vi "lockin ID.vi"(5 "Addresses IN":refnum<visa-resource-name>[](array[refnum]), 7 "names in":string[](array[string]), 8 "error in (no error)":errorcluster, 9 "Lockin address":string, 10 "Lockin on":bool, 11 "Lockin Chan name":string) -> (0 "error out":errorcluster, 2 "Addresses out":refnum<visa-resource-name>[](array[refnum]), 3 "names out":string[](array[string]))   [LabVIEW 2024]
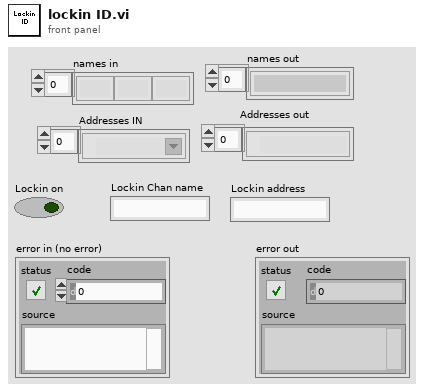
[diagram p1: front panel]
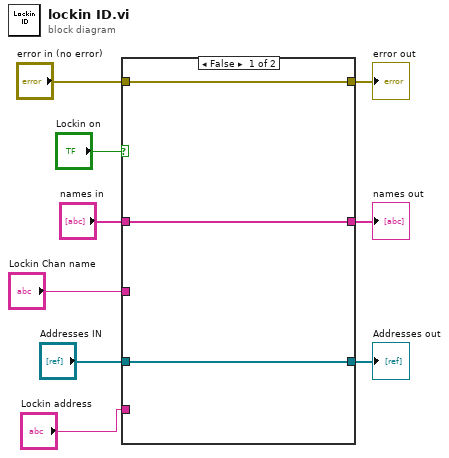
[diagram p0: block diagram]
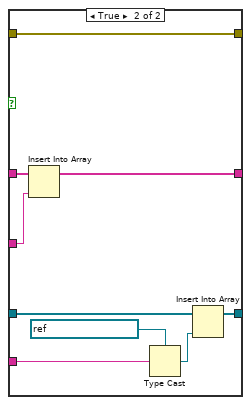
[diagram p2: hidden frame]
diagram:
  n1 = case shown="False" "Lockin on" {
    tunnel: "error in (no error)" -> [w12 w21]
    tunnel: [w12 w21] -> w5
    tunnel: [w11 w13] -> w6
    tunnel: [w10 w16] -> w7
    tunnel: "Lockin Chan name" -> [_ w17]
    tunnel: "Lockin address" -> [_ w19]
    tunnel: "names in" -> [w10 w18]
    tunnel: "Addresses IN" -> [w11 w15]
    frame False {
    }
    frame True {
      n2 = Insert Into Array(array=w18, new element=w17) -> (w16:string[])  [unwired: 1 in]
      n3 = Type Cast(type=refnum<visa-resource-name> "GPIB0::8::INSTR" ("Lockin address 1"), x=w19) -> (*(type *) &x=w14:refnum<visa-resource-name>)
      n4 = Insert Into Array(array=w15, new element=w14) -> (w13:refnum<visa-resource-name>[])  [unwired: 1 in]
    }
  }
  "names out" <- w7
  "Addresses out" <- w6
  "error out" <- w5
